vi "IMA Add DC Point.vi"(0 "WFDC Notifier":refnum<notifier>, 7 "WFDC External Sync":refnum<notifier>, 11 "Error":errorcluster) -> (4 "Scan Path":path, 8 "Canceled":bool, 15 "Error Out":errorcluster)   [LabVIEW 2020]
uses:
  Wide Field Drift Correction/WFDC Controls/WFDC External Sync.ctl
  Wide Field Drift Correction/WFDC Controls/WFDC Cycle Pause.ctl
  Wide Field Drift Correction/WFDC Controls/WFDC Status.ctl
  Wide Field Drift Correction/WFDC Controls/WFDC Notifier Element.ctl
  Wide Field Drift Correction/WFDC Controls/WFDC Actions.ctl
  <vilib>/vision/Image Controls.llb/IMAQ Image.ctl
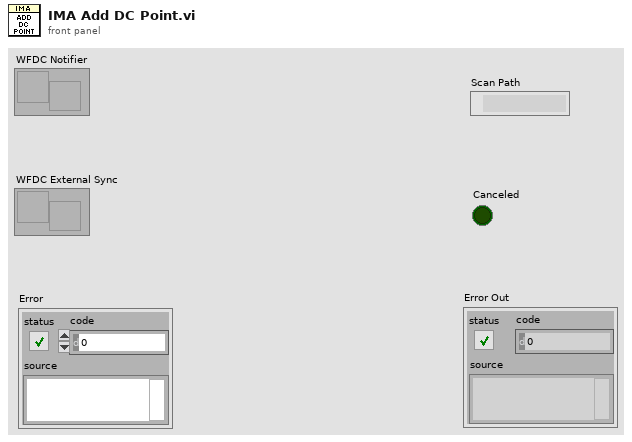
[diagram p1: front panel]
types:
  T1 = typedef "WFDC Actions.ctl" = enum16{"Error Check", "Remote Start", "Move to Pos", "Pre Start Get Drift", "Pre Start Check Drift", "Pre Start Z Drift", "Pre Start XY Drift", "Pre Start ReFocus", "Setup New DC", "Setup Camera", "Get Ref Images", "Calc Calibration", "Switch Tabs", "Get Drift", "Z Drift", "XY Drift", "Start Cycle", "Stop DC", "Abort Remote", "Exit Loop", "Set Error", "Generate Calibration", "Quit"}
  T2 = typedef "WFDC Notifier Element.ctl" = cluster{"WFDC Actions":T1, "Initial XYZ Positions":dbl[], "Ref Images":T3[], "Calibration (slope, inter)":dbl[], "Base Path":path, "Latest Scan Path":path, "Error":errorcluster, "XYZ Drift":dbl[]}
  T3 = typedef "IMAQ Image.ctl" = refnum<image>
  T4 = typedef "WFDC Status.ctl" = enum16{"Idle", "Busy", "DC Active", "Error", "Canceled"}
  T5 = typedef "WFDC External Sync.ctl" = cluster{"Cycle Sync":T6, "Z Offset":dbl, "WFDC Status":T4}
  T6 = typedef "WFDC Cycle Pause.ctl" = enum16{"Pause Requested", "Paused", "Resume Requested", "Resumed"}
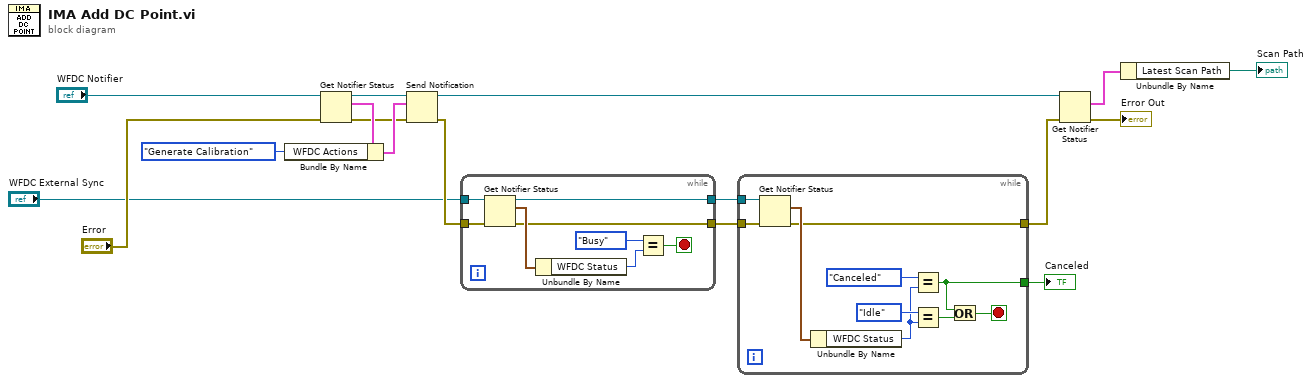
[diagram p0: block diagram]
diagram:
  n1 = Get Notifier Status(notifier="WFDC Notifier", error in (no error)="Error") -> (notifier out=w15:refnum<notifier>, current notification=w14:T2, error out=w10:errorcluster)  [unwired: 2 out]
  n2 = Bundle By Name(cluster=w14, "WFDC Actions"=WFDC_Actions."Generate Calibration") -> (w17:T2)
  n3 = Send Notification(notification=w17, notifier=w15, error in (no error)=w10) -> (notifier out=w13:refnum<notifier>, error out=w7:errorcluster)
  n4 = while {
    tunnel: "WFDC External Sync" -> [w24]
    tunnel: [w20] -> w8
    tunnel: w7 -> [w19]
    tunnel: [w18] -> w6
    stop <- w21 stop-if-true
    n5 = Get Notifier Status(notifier=w24, error in (no error)=w19) -> (notifier out=w20:refnum<notifier>, current notification=w25:T5, error out=w18:errorcluster)  [unwired: 2 out]
    n6 = Unbundle By Name(w25) -> ("WFDC Status"=w23:T4)
    n7 = Equal?(x=WFDC_Status."Busy", y=w23) -> (x = y?=w21:bool)
  }
  n8 = while {
    tunnel: w8 -> [w34]
    tunnel: w6 -> [w33]
    tunnel: [w32] -> w5
    tunnel: [w26] -> w1
    stop <- w27 stop-if-true
    n9 = Get Notifier Status(notifier=w34, error in (no error)=w33) -> (current notification=w35:T5, error out=w32:errorcluster)  [unwired: 3 out]
    n10 = Unbundle By Name(w35) -> ("WFDC Status"=w30:T4)
    n11 = Equal?(x=WFDC_Status."Canceled", y=w30) -> (x = y?=w26:bool)
    n12 = Equal?(x=WFDC_Status."Idle", y=w30) -> (x = y?=w28:bool)
    n13 = Or(x=w26, y=w28) -> (x .or. y?=w27:bool)
  }
  "Canceled" <- w1
  n14 = Get Notifier Status(notifier=w13, error in (no error)=w5) -> (current notification=w12:T2, error out=→"Error Out":errorcluster)  [unwired: 3 out]
  n15 = Unbundle By Name(w12) -> ("Latest Scan Path"=→"Scan Path":path)
